vi "WaveFormMaxMinDecimate.vi"(6 "Plot interpolation":T1(ring)=enum."Average", 8 "error in (no error)":errorcluster, 9 "Total points to remain":i64, 10 "decimation factor":i32=1, 11 "Data in":waveform(sgl)[](array[waveform])) -> (0 "error out":errorcluster, 3 "Data out":waveform(sgl)[](array[waveform]))   [LabVIEW 2015]
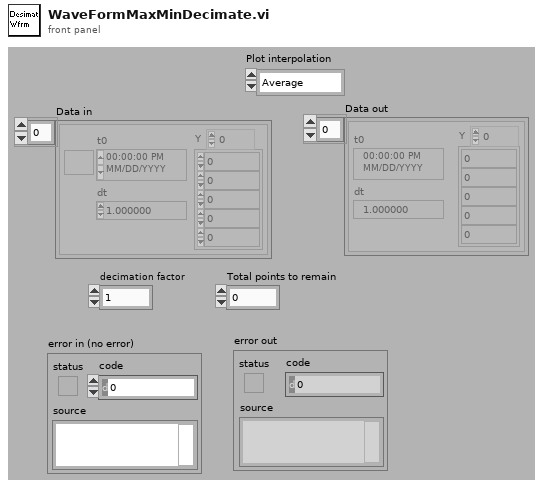
[diagram p1: front panel]
types:
  T1 = enum16{"coerce", "linear", "spline", "Min-Max", "Average"}
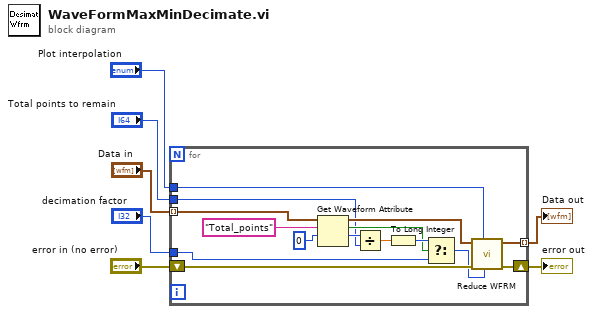
[diagram p0: block diagram]
diagram:
  n1 = for {
    tunnel: "Data in" -> [w22] mode=indexing
    tunnel: "decimation factor" -> [w13]
    tunnel: [w21] -> w5 mode=indexing
    tunnel: "Plot interpolation" -> [w20]
    shift-right: [w16] -> w2
    shift-left: "error in (no error)" -> [w19]
    tunnel: "Total points to remain" -> [w10]
    n2 = Get Waveform Attribute(5:i64 0, 6:"Total_points" ("name"), 7:w22) -> (1:w11:i64, 2:w12:bool, 3:w15:waveform(sgl))  [unwired: 1 in, 1 out]
    n3 = Divide(x=w11, y=w10) -> (x/y=w9:dbl)
    n4 = To Long Integer(number=w9) -> (32bit integer=w14:i32)
    n5 = Select(t=w14, s=w12, f=w13) -> (s? t:f=w8:i32)
    n6 = call "Reduce WFRM.vi"("decimation factor"=w8, "Decimation method"=w20, "error in (no error)"=w19, "Waveform"=w15) -> ("error out"=w16:errorcluster, "Waveform out"=w21:waveform(sgl))  [unwired: 6 in]
  }
  "Data out" <- w5
  "error out" <- w2
